vi "Read From String Delimiter.vi"(8 "error in (no error)":errorcluster, 11 "Array in":refnum<class "Array.lvclass">) -> (0 "error out":errorcluster, 2 "Delimiter":string, 3 "Array out":refnum<class "Array.lvclass">)   [LabVIEW 2019, in "Array.lvclass"]
uses:
  LV_Abstract/Source/Abs_Types/Interfaces/Array/Array.lvclass
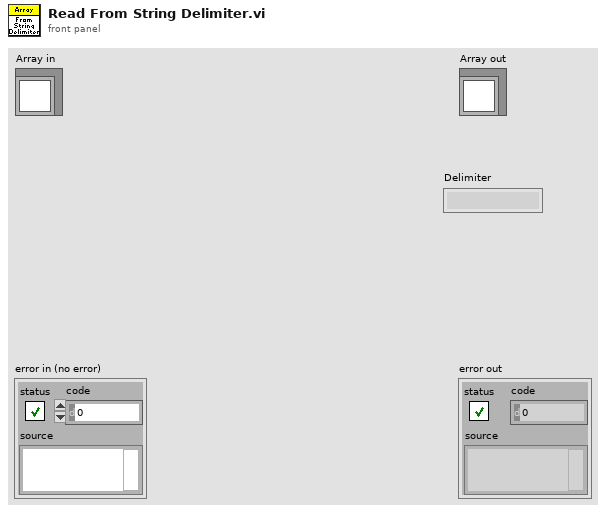
[diagram p1: front panel]
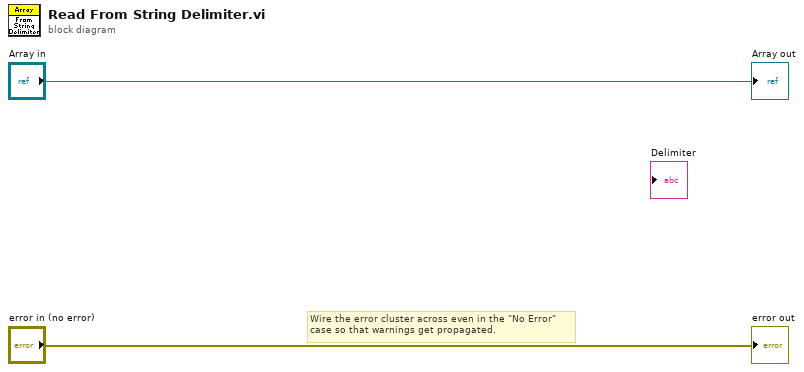
[diagram p0: block diagram]
diagram:
  # "Wire the error cluster across even in the \"No Error\"\ncase so that warnings get propagated."
  "error out" <- "error in (no error)"
  "Array out" <- "Array in"
